vi "Equal.vi"(1 "y":refnum<class "Generic Comparer.lvclass">, 2 "x":refnum<class "Generic Comparer.lvclass">) -> (0 "equal?":bool)   [LabVIEW 2023, in "Generic Comparer.lvclass"]
doc: "Returns TRUE if the value of <b>x</b> is equal to the value of <b>y</b>."
uses:
  Generic Comparer.lvclass
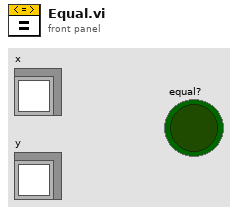
[diagram p1: front panel]
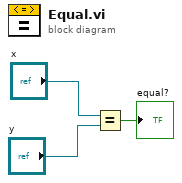
[diagram p0: block diagram]
diagram:
  n1 = Equal?(x="x", y="y") -> (x = y?=→"equal?":bool)
